vi "Concatenate all PDF files.vi"(0 "PDF Report IN":refnum<class "PDF Report Class.lvclass">, 11 "error in (no error)":errorcluster, 12 "Last PageNumber":i32, 13 "TOC page":cluster{"Start":i32, "Number":i32}) -> (4 "PDF Report OUT":refnum<class "PDF Report Class.lvclass">, 15 "error out":errorcluster)   [LabVIEW 2020, in "Exaprom PDF.lvlib"]
doc: "Version 2.0\nDeveloped by Jean-Marc Simard\nCopyright © 2012, Exaprom Inc.\nAll rights reserved.\nLicense: BSD\n\nWith iTextSharp Library\n(http://itextsharp.sourceforge.net)"
uses:
  <userlib>/labview-PDF-writer-master/Exaprom PDF.lvlib
  <userlib>/labview-PDF-writer-master/LV Class/PDF Report Class/PDF Report Class.lvclass
  <userlib>/labview-PDF-writer-master/Controls/General Controls/Create or close.ctl
  <userlib>/labview-PDF-writer-master/Controls/File Path Controls/Temporary File.ctl
panel:
  # "最后一页数量"
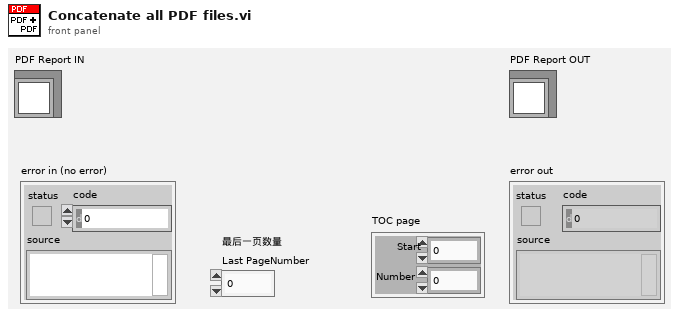
[diagram p1: front panel]
types:
  T1 = typedef "Exaprom PDF.lvlib/Temporary File.ctl" = enum16{".bmp", ".jpeg", ".png", ".pdf", "No File", ".xml"}
  T2 = typedef "Exaprom PDF.lvlib/Create or close.ctl" = enum16{"Create", "Close"}
  T3 = typedef "Exaprom PDF.lvlib/Page dimensions.ctl" = cluster{"Start at page":i32, "Page Size":T4, "Orientation":T5, "widht":sgl, "height":sgl, "Margin left":sgl, "Margin right":sgl, "Margin top":sgl, "Margin bottom":sgl, "X0":sgl, "X1":sgl, "Y0":sgl, "Y1":sgl}
  T4 = typedef "Exaprom PDF.lvlib/Page size.ctl" = i32
  T5 = typedef "Exaprom PDF.lvlib/Page Orientation.ctl" = enum16{"Portrait", "Landscape"}
  T6 = typedef "Exaprom PDF.lvlib/PDF File and position.ctl" = cluster{"Path":path, "Pages":string, "Source":T7, "Start at page old":i32, "Start at page new":i32, "Owner password":string}
  T7 = typedef "Exaprom PDF.lvlib/PDF file source.ctl" = enum16{"PDF Report", "File to add"}
  T8 = typedef "Exaprom PDF.lvlib/File Permission Parameters.ctl" = cluster{"User Password":string, "Owner Password":string, "Printing":enum16{"Allow Printing", "Allow Degraded Printing", "Don't Allow Printing"}, "Allow Modify Contents":bool, "Allow Copy":bool, "Allow Modify Annotations":bool, "Allow Fill In ":bool, "Allow Screen Readers":bool, "Allow Assembly":bool}
  T9 = typedef "Exaprom PDF.lvlib/PDF Details.ctl" = cluster{"Title":string, "Author":string, "Subject":string, "Keywords":string, "Creator":string}
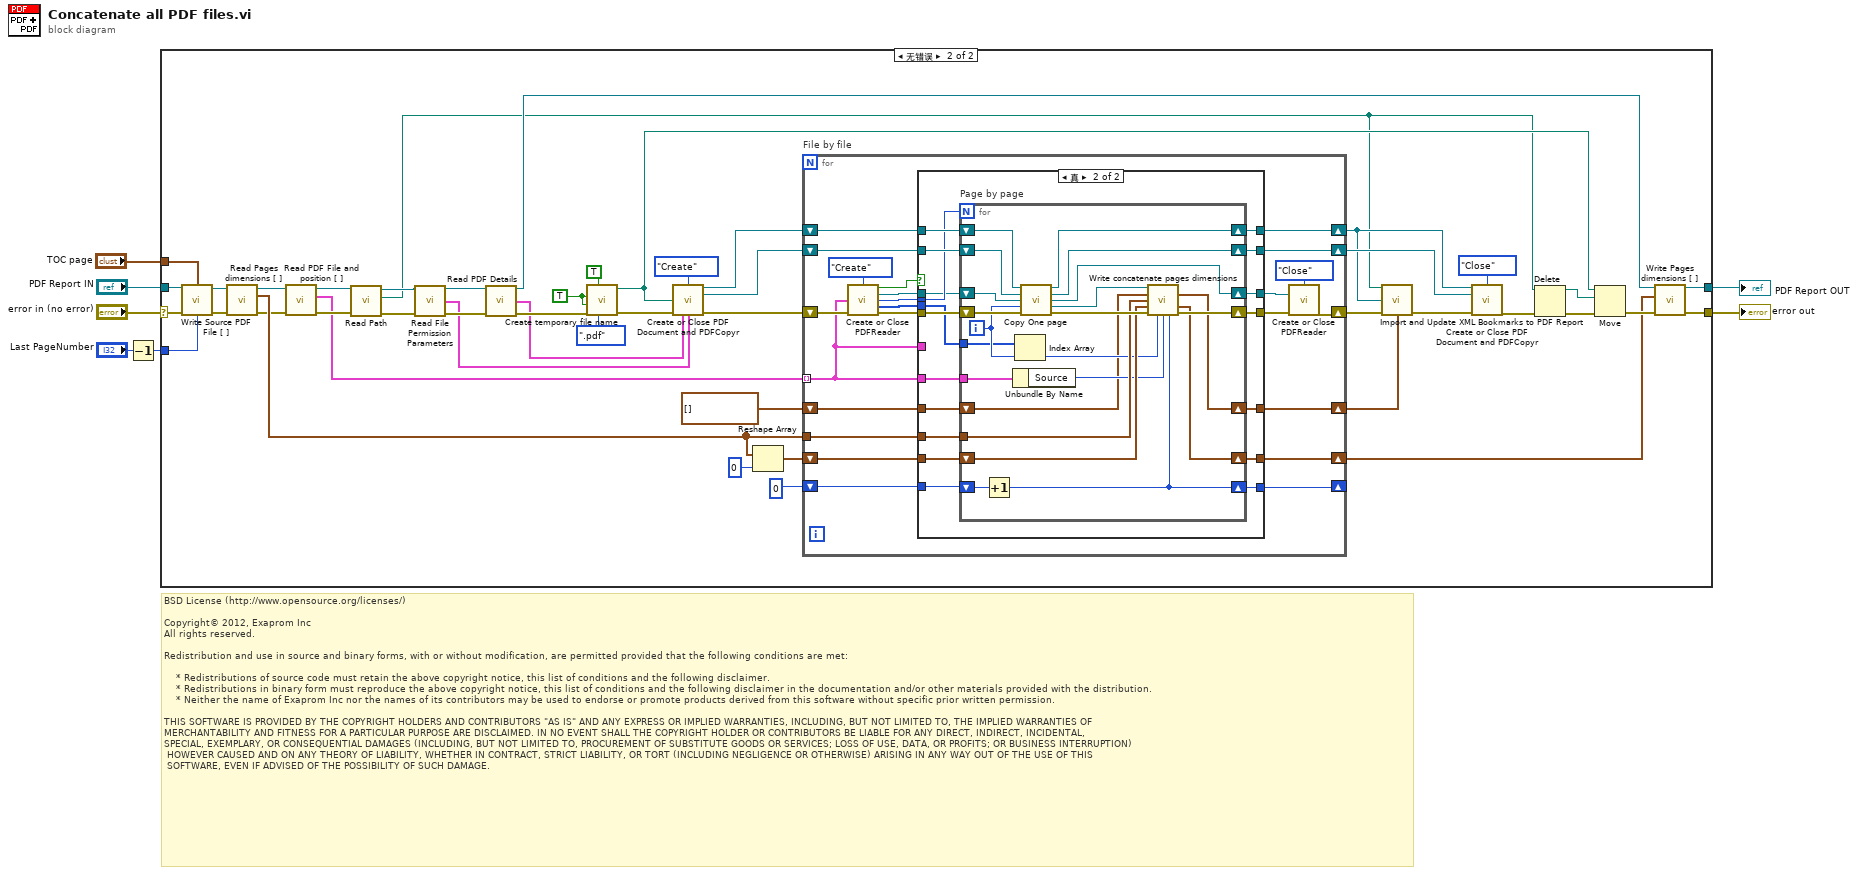
[diagram p0: block diagram]
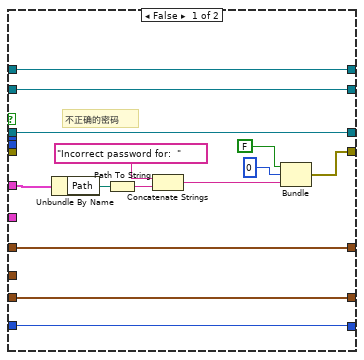
[diagram p3: hidden frame]
diagram:
  # "BSD License (http://www.opensource.org/licenses/)\n\nCopyright© 2012, Exaprom Inc\nAll rights reserved.\n\nRedistribution and use in source and binary forms, with or without modification, are permitted provided that the following conditions are met:\n\n    * Redistributions of source code must retain the above copyright notice, this list of conditions and the following disclaimer.\n    * Redistributions in binary form must reproduce the above copyright notice, this list of conditions and the following disclaimer in the documentation and/or other materials provided with the distribution.\n    * Neither the name of Exaprom Inc nor the names of its contributors may be used to endorse or promote products derived from this software without specific prior written permission.\n\nTHIS SOFTWARE IS PROVIDED BY THE COPYRIGHT HOLDERS AND CONTRIBUTORS \"AS IS\" AND ANY EXPRESS OR IMPLIED WARRANTIES, INCLUDING, BUT NOT LIMITED TO, THE IMPLIED WARRANTIES OF \nMERCHANTABILITY AND FITNESS FOR A PARTICULAR PURPOSE ARE DISCLAIMED. IN NO EVENT SHALL THE COPYRIGHT HOLDER OR CONTRIBUTORS BE LIABLE FOR ANY DIRECT, INDIRECT, INCIDENTAL,\nSPECIAL, EXEMPLARY, OR CONSEQUENTIAL DAMAGES (INCLUDING, BUT NOT LIMITED TO, PROCUREMENT OF SUBSTITUTE GOODS OR SERVICES; LOSS OF USE, DATA, OR PROFITS; OR BUSINESS INTERRUPTION)\n HOWEVER CAUSED AND ON ANY THEORY OF LIABILITY, WHETHER IN CONTRACT, STRICT LIABILITY, OR TORT (INCLUDING NEGLIGENCE OR OTHERWISE) ARISING IN ANY WAY OUT OF THE USE OF THIS\n SOFTWARE, EVEN IF ADVISED OF THE POSSIBILITY OF SUCH DAMAGE."
  n1 = Decrement(x="Last PageNumber") -> (x-1=w2:i32)
  n2 = case shown="无错误" "error in (no error)" {
    selector: "error in (no error)" -> [w9 w55]
    tunnel: [w9 w40] -> w7
    tunnel: "PDF Report IN" -> [w8 w49]
    tunnel: [w8 w39] -> w4
    tunnel: w2 -> [_ w24]
    tunnel: "TOC page" -> [_ w10]
    frame Error {
    }
    frame No Error {
      w47 = TRUE ("hh:mm:ss (false)")
      n3 = call <userlib>:"Write Source PDF File [ ].vi"("PDF Report IN"=w49, "TOC page"=w10, "error in (no error)"=w55, "Last PageNumber"=w24) -> ("PDF Report OUT"=w33:refnum<class "PDF Report Class.lvclass">, "error out"=w34:errorcluster)  [unwired: 10 in]
      n4 = call-dynamic "Read Pages dimensions [ ].vi"("error in (no error)"=w34, "PDF Report Class in"=w33) -> ("error out"=w28:errorcluster, "Pages dimensions [ ]"=w29:T3[], "PDF Report Class out"=w27:refnum<class "PDF Report Class.lvclass">)  [unwired: 6 in, 1 out]
      n5 = call-dynamic "Read PDF File and position [ ].vi"("error in (no error)"=w28, "PDF Report Class in"=w27) -> ("error out"=w37:errorcluster, "PDF File and position [ ]"=w32:T6[], "PDF Report Class out"=w36:refnum<class "PDF Report Class.lvclass">)  [unwired: 7 in]
      n6 = call-dynamic "Read Path.vi"("error in (no error)"=w37, "PDF Report Class in"=w36) -> ("error out"=w35:errorcluster, "Path"=w11:path, "PDF Report Class out"=w19:refnum<class "PDF Report Class.lvclass">)  [unwired: 7 in]
      n7 = call-dynamic "Read File Permission Parameters.vi"("PDF Report Class in"=w19, "error in (no error)"=w35) -> ("PDF Report Class out"=w20:refnum<class "PDF Report Class.lvclass">, "File Permission Parameters"=w17:T8, "error out"=w23:errorcluster)  [unwired: 11 in]
      n8 = call-dynamic "Read PDF Details.vi"("PDF Report Class in"=w20, "error in (no error)"=w23) -> ("PDF Report Class out"=w18:refnum<class "PDF Report Class.lvclass">, "PDF Details"=w21:T9, "error out"=w22:errorcluster)  [unwired: 11 in]
      n9 = call <userlib>:"Create temporary file name.vi"("Temporary Image File"=Temporary_File.".pdf", "Flush Files (F)"=TRUE, "error in (no error)"=w22, "msec (F)"=w47, "hh:mm:ss (false)"=w47) -> ("error out"=w45:errorcluster, "File path"=w41:path)  [unwired: 1 in, 4 out]
      n10 = call <userlib>:"Create or Close PDF Document and PDFCopyr.vi"("Action"=Create_or_close."Create", "File name"=w41, "error in (no error)"=w45, "PDF Details"=w21, "Permissions"=w17) -> ("PDF Copy OUT"=w54:refnum<k24>, "PDF Document OUT"=w53:refnum<k24>, "error out"=w56:errorcluster)  [unwired: 8 in]
      n11 = Reshape Array(w29, 0 ("dimension size")) -> (w31:T3[])
      n12 = for "File by file" {
        tunnel: w32 -> [w59] mode=indexing
        shift-right: [w77] -> w51
        shift-left: w53 -> [w79]
        shift-right: [w69] -> w15
        shift-left: w56 -> [w74]
        shift-right: [w76] -> w12
        shift-left: w54 -> [w78]
        shift-right: [w65] -> w25
        shift-left: w31 -> [w66]
        shift-right: [w63] -> _
        shift-left: 0 ("Page number") -> [w64]
        tunnel: w29 -> [w62]
        shift-right: [w58] -> w13
        shift-left: cluster{"Old":i32, "New":i32}[] [] ("Pages [ ] OUT") -> [w57]
        n13 = call <userlib>:"Create or Close PDFReader.vi"("Action"=Create_or_close."Create", "PDF File and position"=w59, "error in (no error)"=w74) -> ("PDFReaderIsOpen?"=w60:bool, "PdfReader OUT"=w72:refnum<k24>, "NumberOfPages"=w73:i32, "Page [ ]"=w61:i32[], "error out"=w75:errorcluster)  [unwired: 8 in]
        n14 = case shown="真" w60 {
          tunnel: w79 -> [w92 w111]
          tunnel: w78 -> [w93 w110]
          tunnel: [w92 w109] -> w77
          tunnel: [w93 w108] -> w76
          tunnel: w75 -> [_ w107]
          tunnel: w73 -> [_ w106]
          tunnel: w72 -> [w91 w105]
          tunnel: [w81 w104] -> w71
          tunnel: [w91 w103] -> w70
          tunnel: w66 -> [w90 w102]
          tunnel: [w90 w101] -> w65
          tunnel: w64 -> [w89 w100]
          tunnel: [w89 w99] -> w63
          tunnel: w59 -> [_ w98]
          tunnel: w62 -> [_ w97]
          tunnel: w61 -> [_ w96]
          tunnel: w59 -> [w88 _]
          tunnel: [w80 w95] -> w58
          tunnel: w57 -> [w80 w94]
          frame False {
            # "不正确的密码"
            n15 = Unbundle By Name(w88) -> ("Path"=w86:path)
            n16 = Path To String(path=w86) -> (string=w85:string)
            n17 = Concatenate Strings("Incorrect password for:  ", w85) -> (w82:string)
            n18 = Bundle("status"=FALSE, "code"=0, w82) -> (w81:cluster{"status":bool, "code":i32, string})  [unwired: 1 in]
          }
          frame True {
            n19 = for "Page by page" {
              N: w106 -> [_]
              shift-right: [w126] -> w109
              shift-left: w111 -> [w131]
              shift-right: [w125] -> w103
              shift-left: w105 -> [w132]
              shift-right: [w124] -> w104
              shift-left: w107 -> [w133]
              shift-right: [w127] -> w108
              shift-left: w110 -> [w130]
              shift-right: [w119] -> w101
              shift-left: w102 -> [w120]
              shift-right: [w117] -> w99
              shift-left: w100 -> [w129]
              tunnel: w98 -> [w122]
              tunnel: w97 -> [w121]
              tunnel: w96 -> [w115]
              shift-right: [w113] -> w95
              shift-left: w94 -> [w112]
              i -> [w116]
              n20 = Increment(x=w129) -> (x+1=w117:i32)
              n21 = Unbundle By Name(w122) -> ("Source"=w118:T7)
              n22 = Index Array(array=w115, index=w116) -> (element=w114:i32)
              n23 = call <userlib>:"Copy One page.vi"("PDFCopy IN"=w130, "PDF Document IN"=w131, "PdfReader IN"=w132, "index"=w116, "error in (no error)"=w133) -> ("PDFCopy OUT"=w127:refnum<k24>, "PDF Document OUT"=w126:refnum<k24>, "PdfReader OUT"=w125:refnum<k24>, "GetPageSizeWithRotation"=w123:refnum<k24>, "error out"=w128:errorcluster)  [unwired: 6 in]
              n24 = call <userlib>:"Write concatenate pages dimensions.vi"("PageSizeWithRotation"=w123, "Pages [ ] IN"=w112, "Pages dimensions [ ] IN original"=w121, "Pages dimensions [ ] IN"=w120, "error in (no error)"=w128, "Old Page number"=w114, "PDF file source"=w118, "Actual Page number"=w117) -> ("Pages [ ] OUT"=w113:cluster{"Old":i32, "New":i32}[], "Pages dimensions OUT [ ]"=w119:T3[], "error out"=w124:errorcluster)  [unwired: 4 in, 1 out]
            }
          }
        }
        n25 = call <userlib>:"Create or Close PDFReader.vi"("Action"=Create_or_close."Close", "PdfReader IN"=w70, "error in (no error)"=w71) -> ("error out"=w69:errorcluster)  [unwired: 8 in, 4 out]
      }
      n26 = call <userlib>:"Import and Update XML Bookmarks to PDF Report.vi"("PDF path file"=w11, "PDFCopy"=w12, "error in (no error)"=w15, "Pages [ ] OUT"=w13) -> ("error out"=w14:errorcluster)  [unwired: 11 in]
      n27 = call <userlib>:"Create or Close PDF Document and PDFCopyr.vi"("PDF Copy IN"=w12, "Action"=Create_or_close."Close", "PDF Document IN"=w51, "error in (no error)"=w14) -> ("error out"=w42:errorcluster)  [unwired: 9 in, 2 out]
      n28 = Delete(path (use dialog)=w11, error in=w42) -> (deleted path=w44:path, error out=w43:errorcluster)  [unwired: 4 out]
      n29 = Move(source path=w41, error in=w43, 10:w44) -> (error out=w26:errorcluster)  [unwired: 4 out]
      n30 = call-dynamic "Write Pages dimensions [ ].vi"("error in (no error)"=w26, "Pages dimensions [ ]"=w25, "PDF Report Class in"=w18) -> ("error out"=w40:errorcluster, "PDF Report Class out"=w39:refnum<class "PDF Report Class.lvclass">)  [unwired: 7 in]
    }
  }
  "error out" <- w7
  "PDF Report OUT" <- w4
